vi "ATF-Globals.vi"() -> ()   [LabVIEW 2022 SP3]
panel:
  out "EXIT":bool
  out "Stop Daq":bool
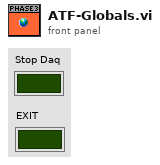
[diagram p1: front panel]
diagram:
